vi "View Log.vi"(8 "error in":errorcluster, 11 "file path":path) -> (0 "error out":errorcluster)   [LabVIEW 2021]
uses:
  <vilib>/Utility/file.llb/Read Delimited Spreadsheet (string).vi
panel:
  in  "OK":bool
  out "Table":string[][](table)
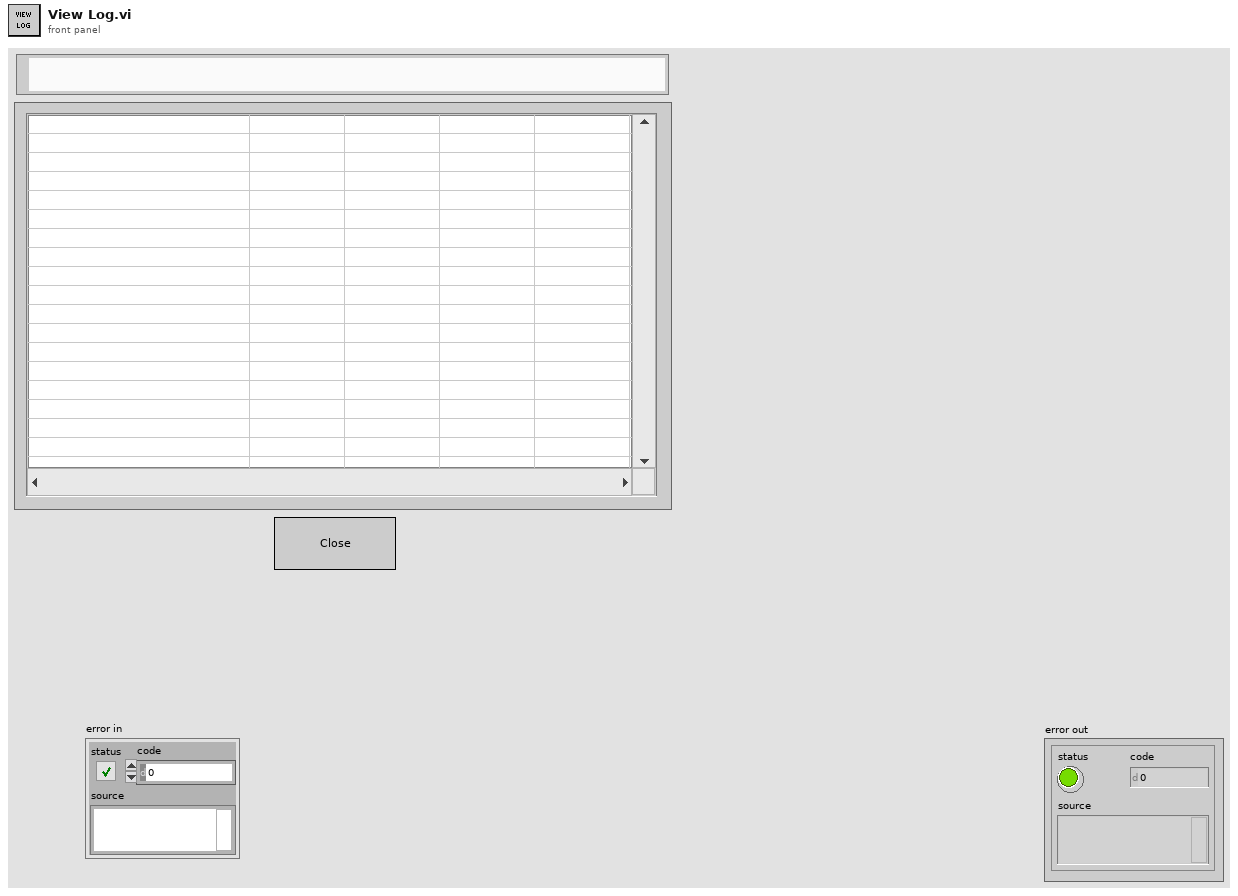
[diagram p1: front panel]
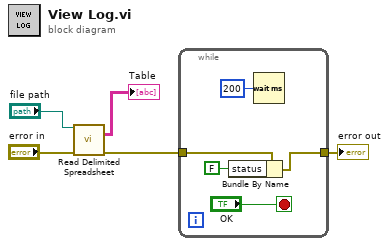
[diagram p0: block diagram]
diagram:
  n1 = call-poly <vilib>:"Read Delimited Spreadsheet.vi"("file path (dialog if empty)"="file path", "error in (no error)"="error in") -> ("all rows"=→"Table":string[][], "error out"=w4:errorcluster)  [unwired: 8 in, 4 out]
  n2 = while {
    tunnel: w4 -> [w8]
    tunnel: [w7] -> w2
    stop <- "OK" stop-if-true
    n3 = Bundle By Name(cluster=w8, "status"=FALSE) -> (w7:errorcluster)
    n4 = Wait (ms)(milliseconds to wait=u32 200) -> ()  [unwired: 1 out]
  }
  "error out" <- w2
